vi "Subscribe to Results.vi"(8 "error in (no error)":errorcluster, 10 "Result Observer":refnum<class "Result Observer.lvclass">, 11 "Parallell Test Runner In":refnum<class "Parallell Test Runner.lvclass">) -> (0 "error out":errorcluster, 3 "Parallell Test Runner Out":refnum<class "Parallell Test Runner.lvclass">)   [LabVIEW 2020, in "Parallell Test Runner.lvclass"]
uses:
  Parallell Test Runner.lvclass
  Result Observer/Result Observer.lvclass
  Parallell Test Runner.lvclass/Parallell Test Runner.ctl
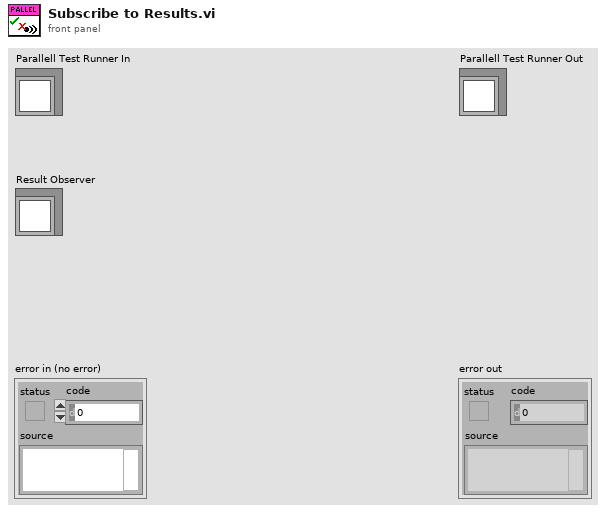
[diagram p1: front panel]
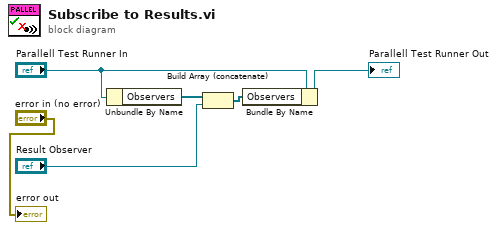
[diagram p0: block diagram]
diagram:
  n1 = Unbundle By Name("Parallell Test Runner In") -> ("Observers"=w4:refnum<class "Result Observer.lvclass">[])
  n2 = Build Array (concatenate)(w4, "Result Observer") -> (w1:refnum<class "Result Observer.lvclass">[])
  n3 = Bundle By Name(cluster="Parallell Test Runner In", "Observers"=w1) -> (→"Parallell Test Runner Out":refnum<class "Parallell Test Runner.lvclass">)
  "error out" <- "error in (no error)"
